vi "oax_Config DSA Channel (MCM).vi"(0 "DAQ Config":T5 {"probe angle [deg]" max=360; "pregain" format="%.2f"; "IEPE" items=["On", "Off", "None"]; "coupling" items=["DC", "AC"]; "engineering units" items=["custom..."=0, "V"=1, "A"=21, "C"=30, "pC"=31, "s"=32, "-"=29, "Pa"=2, "N"=20, "g"=3, "m/s^2"=4, "m/s"=5, "m"=6, "mm/s"=12, "mm"=13, "micron/s"=14, "micron"=15, "in/s^2"=7, "in/s"=8, "in"=9, "mil/s"=10, "mil"=11, "rad/s^2"=16, "rad/s"=17, "rad"=18, "deg/s^2"=26, "deg/s"=27, "deg"=28, "RPM"=22, "cycle/s^2"=23, "Hz"=24, "cycle"=25, "strain"=19]; "sensor sensitivity (mV/EU)" format="%.2f"; "dB reference" format="%.1e"}, 1 "tachometer channel":tag, 5 "error in (no error)":errorcluster, 6 "sample rate [samples/s]":dbl=10000.0, 7 "rotating direction":u16(ring) items=["CCW", "CW"], 8 "max value":dbl=5.0 format="%0.2f", 10 "min value":dbl=-5.0 format="%0.2f") -> (11 "channel name":string[](array[string]), 13 "channel info":T2[](array[typedef]) {"pregain" format="%.2f"; "weighting filter" items=["Linear", "A-weighting", "B-weighting", "C-weighting", "ITU-R 468-4", "Dolby", "CCITT", "C-message", "Wb", "Wc", "Wd", "We", "Wf", "Wh", "Wj", "Wk", "Wm", "AES17 20 kHz lowpass", "AES17 40 kHz lowpass", "AES17 20 kHz highpass", "AES17 40 kHz highpass"]; "dB reference" format="%^.1e"; "engineering units" items=["custom..."=0, "V"=1, "A"=21, "C"=30, "pC"=31, "s"=32, "-"=29, "Pa"=2, "N"=20, "g"=3, "m/s^2"=4, "m/s"=5, "m"=6, "mm/s"=12, "mm"=13, "micron/s"=14, "micron"=15, "in/s^2"=7, "in/s"=8, "in"=9, "mil/s"=10, "mil"=11, "rad/s^2"=16, "rad/s"=17, "rad"=18, "deg/s^2"=26, "deg/s"=27, "deg"=28, "RPM"=22, "cycle/s^2"=23, "Hz"=24, "cycle"=25, "strain"=19]; "sensor sensitivity" format="%#_5f"}, 14 "task out":refnum<k21>, 15 "tacho channel index":i32, 18 "channel properties":T1[](array[typedef]) {"probe angle [deg]" max=360; "direction" items=["CCW", "CW"]}, 19 "error out":errorcluster)   [LabVIEW 2017]
doc: "Configures DAQ channel properties based on the user input and starts the DAQmx task."
uses:
  <vilib>/addons/Sound and Vibration/Order Analysis/Example Support/sub VIs/OAXML_DSA MCM DAQ Config.ctl
  <vilib>/addons/_NISVFA/_Shared subVIs/Controls/svc_Engineering Units Text Ring.ctl
  <vilib>/addons/_NISVFA/_Shared subVIs/Controls/svc_Channel Info.ctl
  <vilib>/addons/_NISVFA/_Shared subVIs/Controls/svc_Weighting Filter Text Ring.ctl
  <vilib>/addons/Sound and Vibration/Order Analysis/Data Presentation/SubVIs/OAT MCM Channel Property.ctl
  <vilib>/DAQmx/configure/timing.llb/DAQmx Timing (Sample Clock).vi
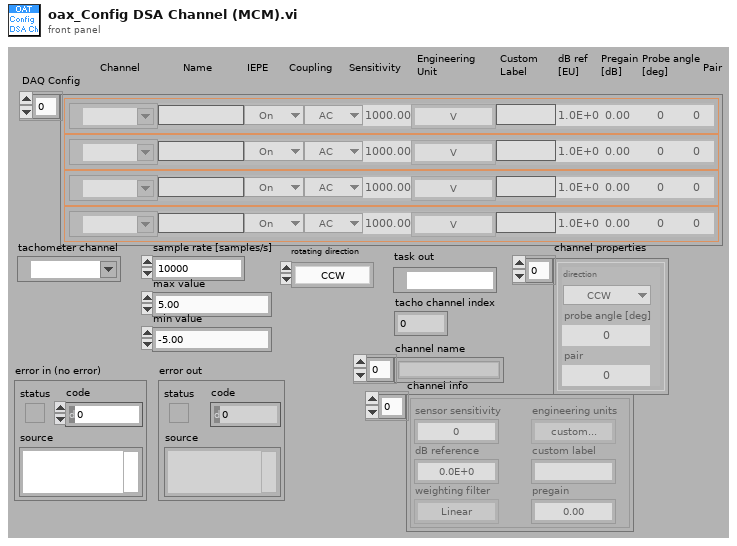
[diagram p1: front panel]
types:
  T1 = typedef "OAT MCM Channel Property.ctl" = cluster{"direction":u16, "probe angle [deg]":u16, "pair":u16}
  T2 = typedef "svc_Channel Info.ctl" = cluster{"sensor sensitivity":dbl, "engineering units":T3, "dB reference":dbl, "custom label":string, "weighting filter":T4, "pregain":dbl}
  T3 = typedef "svc_Engineering Units Text Ring.ctl" = u16
  T4 = typedef "svc_Weighting Filter Text Ring.ctl" = u16
  T5 = typedef "OAXML_DSA MCM DAQ Config.ctl" = cluster{"name":string, "channel":tag, "coupling":u16, "dB reference":sgl, "sensor sensitivity (mV/EU)":dbl, "engineering units":T3, "IEPE":u16, "custom label":string, "pregain":sgl, "probe angle [deg]":u16, "pair":u16}[]
  T6 = typedef "OAXML_DSA DAQ Config.ctl" = cluster{"name":string, "channel":tag, "coupling":u16, "dB reference":sgl, "sensor sensitivity (mV/EU)":dbl, "engineering units":T3, "IEPE":u16, "custom label":string, "pregain":sgl}[]
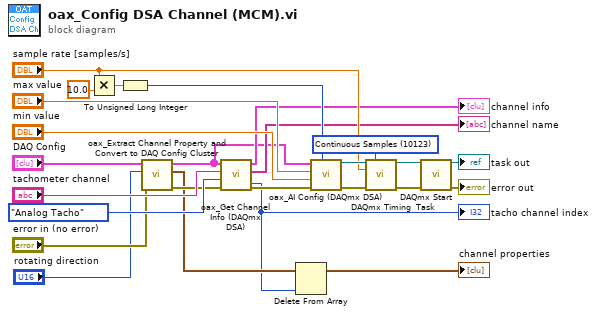
[diagram p0: block diagram]
diagram:
  w22 = 10123 items=["Finite Samples"=10178, "Continuous Samples"=10123, "Hardware Timed Single Point"=12522] ("sample mode")
  n1 = Multiply(x="sample rate [samples/s]", y=10.0) -> (x*y=w16:dbl)
  n2 = To Unsigned Long Integer(number=w16) -> (unsigned 32bit integer=w13:u32)
  n3 = call <vilib>:"oax_Extract Channel Property and Convert to DAQ Config Cluster.vi"("error in (no error)"="error in (no error)", "rotating direction"="rotating direction", "MCM DAQ Config"="DAQ Config") -> ("error out"=w5:errorcluster, "channel properties"=w3:T1[], "DAQ Config"=w7:T6)  [unwired: 6 in]
  n4 = call <vilib>:"oax_Get Channel Info (DAQmx DSA).vi"("error in (no error)"=w5, "Tacho Type"=enum16{"Analog Tacho", "Digital Tacho"}."Analog Tacho", "tachometer channel"="tachometer channel", "DAQ Config"=w7) -> ("error out"=w24:errorcluster, "channel name"=→"channel name":string[], "channel info"=→"channel info":T2[], "tacho channel index"=w1:i32)  [unwired: 2 in, 2 out]
  "tacho channel index" <- w1
  n5 = Delete From Array(array=w3, index=w1) -> (array with subset deleted=→"channel properties":T1[])  [unwired: 1 in, 1 out]
  n6 = call <vilib>:"oax_AI Config (DAQmx DSA).vi"("buffer size"=w13, "error in (no error)"=w24, "min value"="min value", "max value"="max value", "DAQ Config"=w7) -> ("error out"=w25:errorcluster, "task out"=w26:refnum<k21>)  [unwired: 5 in]
  n7 = call-poly <vilib>:"DAQmx Timing.vi"("task/channels in"=w26, "sample mode"=w22, "rate"="sample rate [samples/s]", "error in"=w25) -> ("task out"=w23:refnum<k21>, "error out"=w21:errorcluster)  [unwired: 10 in]
  n8 = call <vilib>:"DAQmx Start Task.vi"("task/channels in"=w23, "error in"=w21) -> ("task out"=→"task out":refnum<k21>, "error out"=→"error out":errorcluster)  [unwired: 12 in]
